vi "G4SubTemplate_Singleton_5x6x5_ReadAttribute.vi"(11 "Error In":errorcluster) -> (15 "Error Out":errorcluster)   [LabVIEW 2020]
uses:
  <resource>/Framework/Providers/Open_GDS/ClassProviders/Provider_EndevoGOOP400/Templates/G4SubTemplate_Singleton_5x6x5/G4SubTemplate_Singleton_5x6x5.lvclass
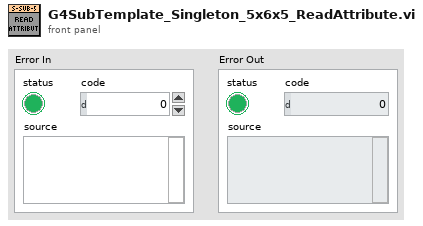
[diagram p1: front panel]
types:
  T1 = typedef "G4SubTemplate_Singleton_5x6x5.lvclass/ObjectAttributes.ctl" = cluster{"Attribute1":dbl}
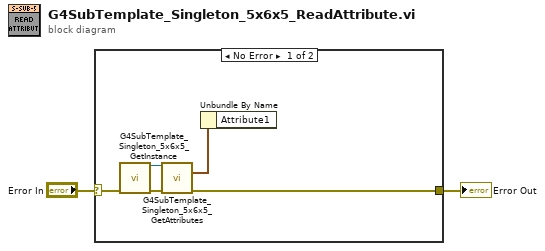
[diagram p0: block diagram]
diagram:
  n1 = case shown="No Error" "Error In" {
    selector: "Error In" -> [w4 w8]
    tunnel: [w6 w8] -> w1
    frame No Error {
      n2 = call <resource>:"G4SubTemplate_Singleton_5x6x5_GetInstance.vi"("Error In"=w4) -> ("reference out"=w5:refnum<class "G4SubTemplate_Singleton_5x6x5.lvclass">, "Error Out"=w3:errorcluster)  [unwired: 10 in, 3 out]
      n3 = call <resource>:"G4SubTemplate_Singleton_5x6x5_GetAttributes.vi"("reference in"=w5, "Error In"=w3) -> ("Data"=w7:T1, "Error Out"=w6:errorcluster)  [unwired: 10 in, 2 out]
      n4 = Unbundle By Name(w7) -> ()  [unwired: 1 out]
    }
    frame Error {
    }
  }
  "Error Out" <- w1
